vi "E3631A Current Setting.vi"(8 "error in (no error)":errorcluster, 9 "Current(A)":dbl format="%.3f", 10 "Channel":i32(ring)=1 items=["Channel 1"=1, "Channel 2"=2, "Channel 3"=3], 11 "VISA resource name":refnum<visa-resource-name>) -> (0 "error out":errorcluster, 3 "VISA resource name out":refnum<visa-resource-name>)   [LabVIEW 2012]
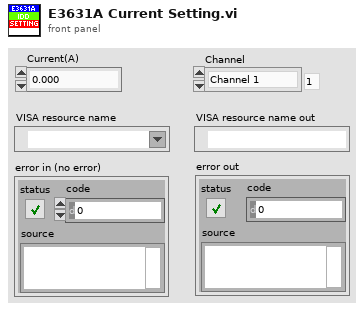
[diagram p1: front panel]
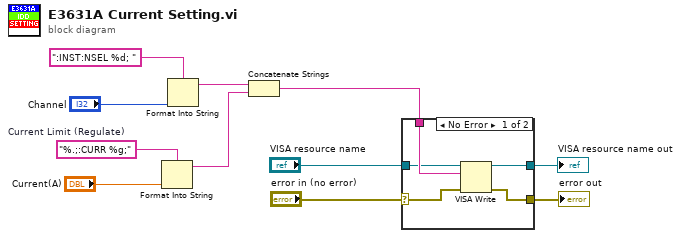
[diagram p0: block diagram]
diagram:
  w7 = "%.;:CURR %g;"  # Current Limit (Regulate)
  n1 = Format Into String(format string=w7, "Current(A)") -> (resulting string=w6:string)  [unwired: 2 in, 1 out]
  n2 = Format Into String(format string=":INST:NSEL %d; ", "Channel") -> (resulting string=w10:string)  [unwired: 2 in, 1 out]
  n3 = Concatenate Strings(w10, w6) -> (w5:string)
  n4 = case shown="No Error" "error in (no error)" {
    selector: "error in (no error)" -> [w12 w18]
    tunnel: w5 -> [w16 _]
    tunnel: "VISA resource name" -> [w15 w17]
    tunnel: [w14 w17] -> w3
    tunnel: [w13 w18] -> w2
    frame No Error {
      n5 = VISA Write(VISA resource name=w15, write buffer=w16, error in (no error)=w12) -> (VISA resource name out=w14:refnum<visa-resource-name>, error out=w13:errorcluster)  [unwired: 1 out]
    }
    frame Error {
    }
  }
  "VISA resource name out" <- w3
  "error out" <- w2
